vi "ini_read_int64_vector.vi"(7 "section":string, 8 "error in":errorcluster, 9 "default":i64[](array[numeric]), 10 "key":string, 11 "refnum in":T1) -> (0 "error out":errorcluster, 1 "values":i64[](array[numeric]), 2 "found?":bool, 3 "refnum out":T1)   [LabVIEW 2018]
uses:
  <vilib>/Utility/config.llb/Config Data RefNum.ctl
  <vilib>/Utility/config.llb/Read Key (String).vi
  <vilib>/Utility/config.llb/NI_LVConfig.lvlib
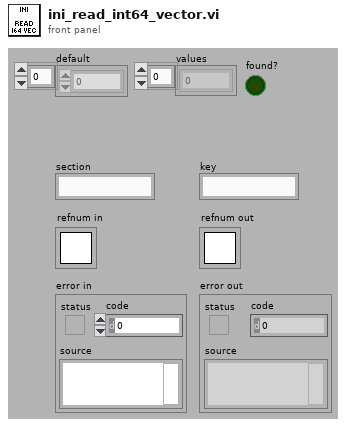
[diagram p1: front panel]
types:
  T1 = typedef "NI_LVConfig.lvlib/Config Data RefNum.ctl" = refnum<k1>
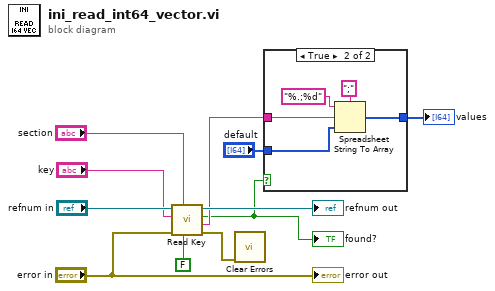
[diagram p0: block diagram]
diagram:
  n1 = call-poly <vilib>:"Read Key.vi"("read raw string? (F)"=FALSE, "section"="section", "error in (no error)"="error in", "key"="key", "refnum"="refnum in") -> ("error out"=w6:errorcluster, "value"=w5:string, "found?"=w4:bool, "refnum out"=→"refnum out":T1)  [unwired: 3 in]
  "found?" <- w4
  n2 = call <vilib>:"Clear Errors.vi"("error in (no error)"=w6) -> ()  [unwired: 5 in, 2 out]
  n3 = case shown="True" w4 {
    tunnel: w5 -> [_ w15]
    tunnel: "default" -> [w12 w14]
    tunnel: [w12 w13] -> w2
    frame False {
    }
    frame True {
      n4 = Spreadsheet String To Array(delimiter (Tab)=";", format string="%.;%d", spreadsheet string=w15, array type (2D Dbl)=w14) -> (array=w13:i64[])
    }
  }
  "values" <- w2
  "error out" <- "error in"
